vi "CRYSet Signal Path Front Panel.vi"(11 "Vi Ref":refnum<vi>) -> ()   [LabVIEW 2013]
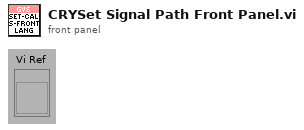
[diagram p1: front panel]
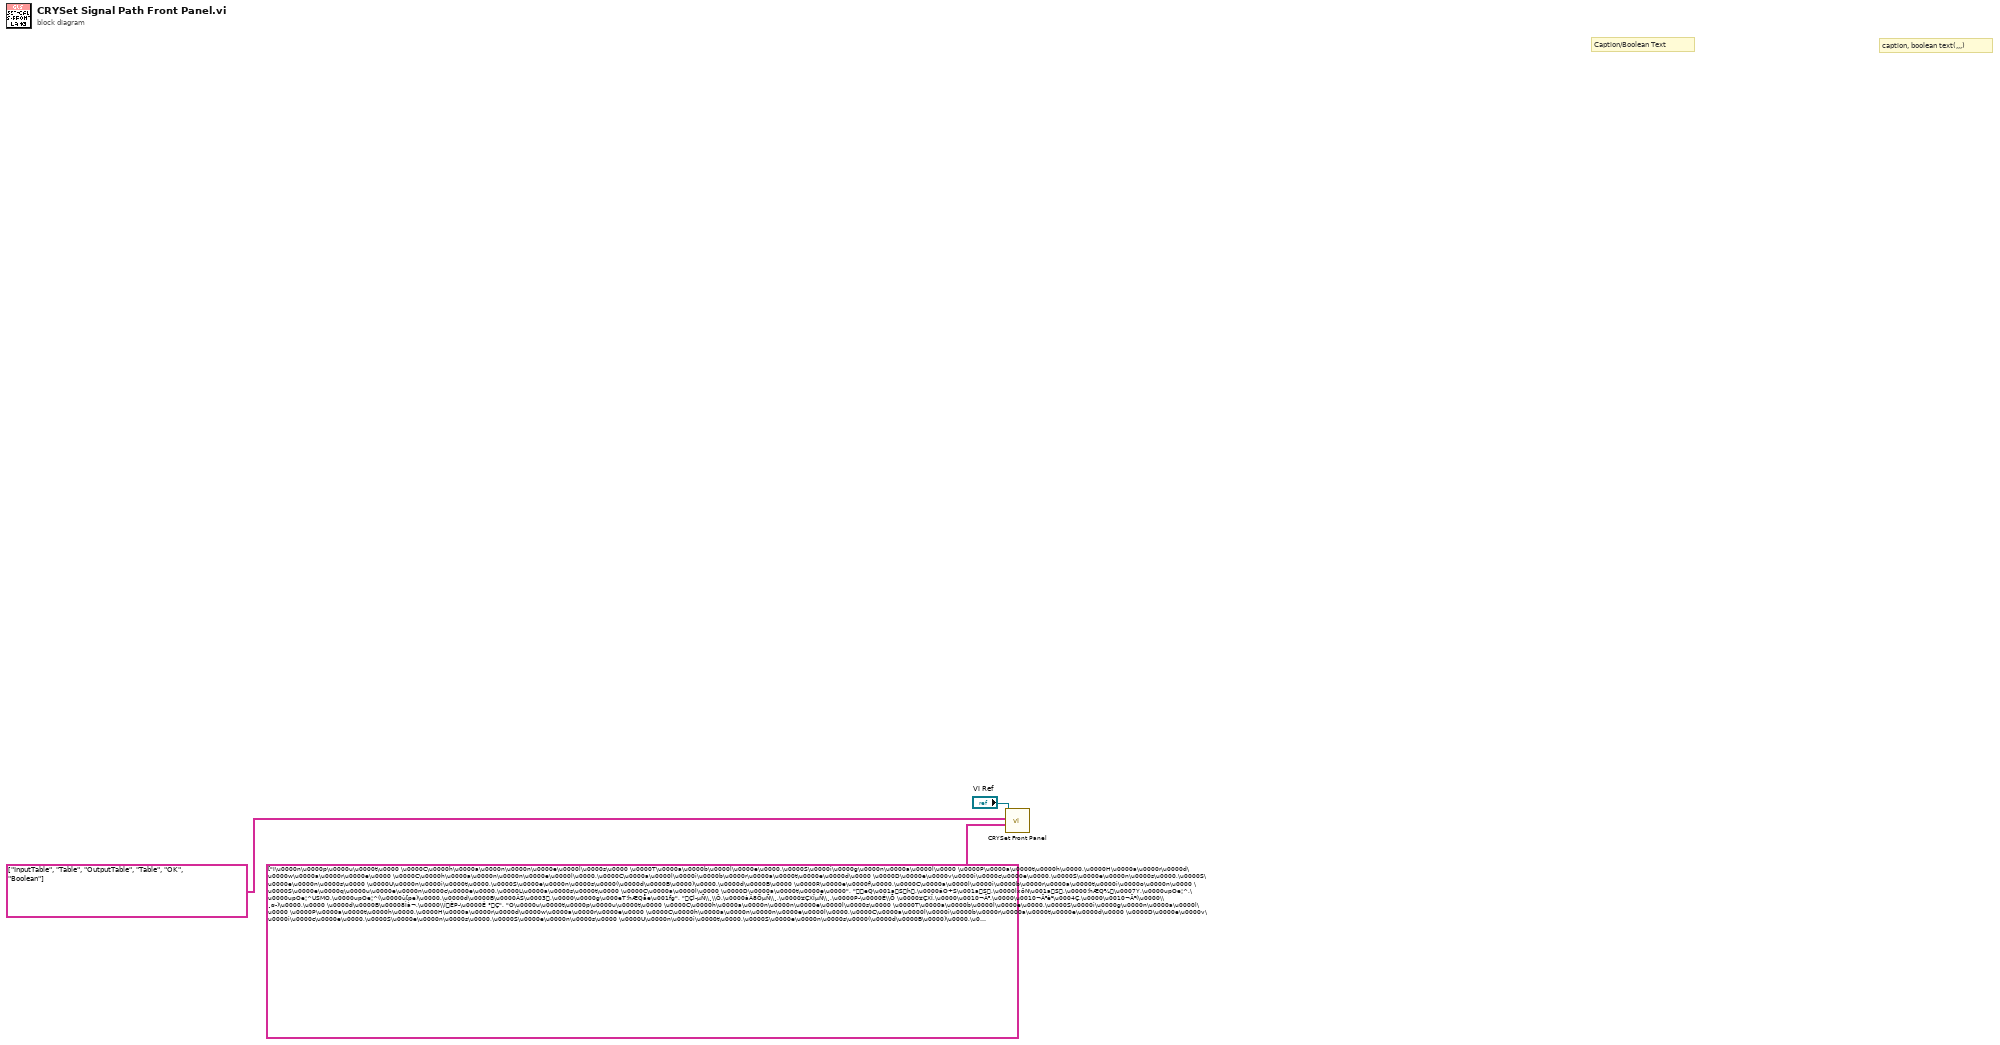
[diagram p0: block diagram]
diagram:
  # "caption, boolean text(,,,)"
  # "Caption/Boolean Text"
  n1 = call "CRYSet Front Panel.vi"("Caption(Boolean Text)"=string[][] [["I\u0000n\u0000p\u0000u\u0000t\u0000 \u0000C\u0000h\u0000a\u0000n\u0000n\u0000e\u0000l\u0000s\u0000 \u0000T\u0000a\u0000b\u0000l\u0000e\u0000,\u0000S\u0000i\u0000g\u0000n\u0000a\u0000l\u0000 \u0000P\u0000a\u0000t\u0000h\u0000,\u0000H\u0000a\u0000r\u0000d\u0000w\u0000a\u0000r\u0000e\u0000 \u0000C\u0000h\u0000a\u0000n\u0000n\u0000e\u0000l\u0000,\u0000C\u0000a\u0000l\u0000i\u0000b\u0000r\u0000a\u0000t\u0000e\u0000d\u0000 \u0000D\u0000e\u0000v\u0000i\u0000c\u0000e\u0000,\u0000S\u0000e\u0000n\u0000s\u0000,\u0000S\u0000e\u0000n\u0000s\u0000 \u0000U\u0000n\u0000i\u0000t\u0000,\u0000S\u0000e\u0000n\u0000s\u0000(\u0000d\u0000B\u0000)\u0000,\u0000d\u0000B\u0000 \u0000R\u0000e\u0000f\u0000,\u0000C\u0000a\u0000l\u0000i\u0000b\u0000r\u0000a\u0000t\u0000i\u0000o\u0000n\u0000 \u0000S\u0000e\u0000q\u0000u\u0000e\u0000n\u0000c\u0000e\u0000,\u0000L\u0000a\u0000s\u0000t\u0000 \u0000C\u0000a\u0000l\u0000 \u0000D\u0000a\u0000t\u0000e\u0000", "eQ\u001aSh,\u0000áO÷S\u001aS,\u0000lxöN\u001aS,\u0000!hÆQ¾\u0007Y,\u0000upOe¦^,\u0000upOe¦^USMO,\u0000upOe¦^(\u0000ù[pe)\u0000,\u0000d\u0000B\u0000ÂS\u0003,\u0000\u0000g\u000eT!hÆQåe\u001fg", "Çl­µÑ\\¸\\Ô,\u0000àÂ8ÖµÑ\\¸,\u0000¥ÇXÎµÑ\\¸,\u0000P­\u0000É\\Õ \u0000¥ÇXÎ,\u0000\u0010¬Ä³,\u0000\u0010¬Ä³è²\u0004Ç,\u0000\u0010¬Ä³(\u0000\\¸ø­)\u0000,\u0000 \u0000d\u0000B\u00008Ìà¬,\u0000\\ÍÈP­\u0000É °Ç"], ["O\u0000u\u0000t\u0000p\u0000u\u0000t\u0000 \u0000C\u0000h\u0000a\u0000n\u0000n\u0000e\u0000l\u0000s\u0000 \u0000T\u0000a\u0000b\u0000l\u0000e\u0000,\u0000S\u0000i\u0000g\u0000n\u0000a\u0000l\u0000 \u0000P\u0000a\u0000t\u0000h\u0000,\u0000H\u0000a\u0000r\u0000d\u0000w\u0000a\u0000r\u0000e\u0000 \u0000C\u0000h\u0000a\u0000n\u0000n\u0000e\u0000l\u0000,\u0000C\u0000a\u0000l\u0000i\u0000b\u0000r\u0000a\u0000t\u0000e\u0000d\u0000 \u0000D\u0000e\u0000v\u0000i\u0000c\u0000e\u0000,\u0000S\u0000e\u0000n\u0000s\u0000,\u0000S\u0000e\u0000n\u0000s\u0000 \u0000U\u0000n\u0000i\u0000t\u0000,\u0000S\u0000e\u0000n\u0000s\u0000(\u0000d\u0000B\u0000)\u0000,\u0000d\u0000B\u0000 \u0000R\u0000e\u0000f\u0000,\u0000C\u0000a\u0000l\u0000i\u0000b\u0000r\u0000a\u0000t\u0000i\u0000o\u0000n\u0000 \u0000S\u0000e\u0000q\u0000u\u0000e\u0000n\u0000c\u0000e\u0000,\u0000L\u0000a\u0000s\u0000t\u0000 \u0000C\u0000a\u0000l\u0000 \u0000D\u0000a\u0000t\u0000e\u0000", "úQ\u001aSh,\u0000áO÷S\u001aS,\u0000lxöN\u001aS,\u0000!hÆQ¾\u0007Y,\u0000upOe¦^,\u0000upOe¦^USMO,\u0000upOe¦^(\u0000ù[pe)\u0000,\u0000d\u0000B\u0000ÂS\u0003,\u0000\u0000g\u000eT!hÆQåe\u001fg", "Íl­µÑ\\¸\\Ô,\u0000àÂ8ÖµÑ\\¸,\u0000¥ÇXÎµÑ\\¸,\u0000P­\u0000É\\Õ \u0000¥ÇXÎ,\u0000\u0010¬Ä³,\u0000\u0010¬Ä³è²\u0004Ç,\u0000\u0010¬Ä³(\u0000\\¸ø­)\u0000,\u0000 \u0000d\u0000B\u00008Ìà¬,\u0000\\ÍÈP­\u0000É °Ç"], ["O\u0000K\u0000", "nx¤‹", "UÖxÇ"]], "Control ID and Type(Label Name, Type)"=string[][] [["InputTable", "Table"], ["OutputTable", "Table"], ["OK", "Boolean"]], "Vi Ref"="Vi Ref") -> ()  [unwired: 9 in]
